vi "tagDB dbChanged.vi"(8 "error in (no error)":errorcluster, 11 "DB Ref":T1) -> (0 "error in (no error) (dup)":errorcluster, 2 "changed?":bool, 3 "DB Ref (dup)":T1)   [LabVIEW 2014, in "TagDB(dev).lvlib"]
uses:
  TagDB(dev).lvlib
  tagDB_Def.ctl
  Private/_Cast TagDB Ref to DVR.vi
  Error/_[error50000]Invalid DB REF.vi
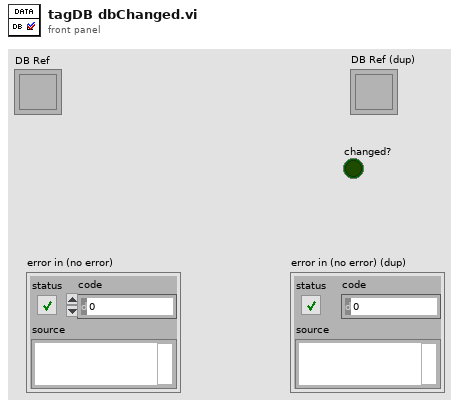
[diagram p1: front panel]
types:
  T1 = typedef "TagDB(dev).lvlib/tagDB_Def.ctl" = refnum<k1>
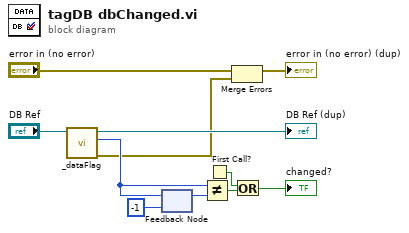
[diagram p0: block diagram]
diagram:
  n1 = call "_dataFlag.vi"("DB Ref"="DB Ref") -> ("error in (no error) (dup)"=w2:errorcluster, "DataChangeFlag"=w3:i64, "DB Ref (dup)"=→"DB Ref (dup)":T1)  [unwired: 8 in]
  n2 = feedback-in #1(w3) -> ()
  n3 = feedback #1(i64 -1 ("DataChangeFlag")) -> (w8:i64)
  n4 = Not Equal?(x=w3, y=w8) -> (x != y?=w7:bool)
  n5 = First Call?() -> (First Call?: T/F=w6:bool)
  n6 = Merge Errors("error in (no error)", w2) -> (→"error in (no error) (dup)":errorcluster)
  n7 = Or(x=w6, y=w7) -> (x .or. y?=→"changed?":bool)
